vi "DIO 1-bit.vi"(8 "DIR":bool, 9 "OUT":bool, 11 "DIO Refnum":refnum<k21>) -> (3 "IN":bool)   [LabVIEW 2013]
uses:
  <vilib>/rvi/eio/common/nirviEmuTemplateMethod_errors.vi
  <vilib>/eio/EIOMethodNode/EIOMethodNode.xnode
  <vilib>/eio/EIONode/EIONode.xnode
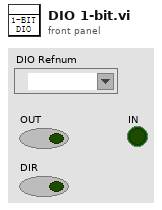
[diagram p1: front panel]
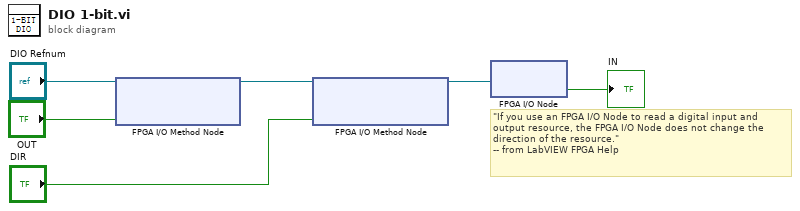
[diagram p0: block diagram]
diagram:
  # "\"If you use an FPGA I/O Node to read a digital input and output resource, the FPGA I/O Node does not change the direction of the resource.\"\n-- from LabVIEW FPGA Help"
  n1 = xnode "FPGA I/O Method Node"("FPGA I/O In"="DIO Refnum", "Data"="OUT") -> ("FPGA I/O Out"=w2:refnum<k21>)
  n2 = xnode "FPGA I/O Method Node"("FPGA I/O In"=w2, "Enable"="DIR") -> ("FPGA I/O Out"=w1:refnum<k21>)
  n3 = xnode "FPGA I/O Node"("FPGA I/O输入"=w1) -> ("I/O项"=→"IN":bool)  [unwired: 1 out]
